vi "Update Data Plot.vi"(6 "Sample Rate (sec/sample)":dbl, 8 "Time interval (s)":i32, 9 "Pump Controller State":T2, 10 "History length (-1; unlimited)":i32=-1, 11 "Graph History Arrays in":T1) -> (0 "Updated Plot History":cluster{timestamp[], dbl[]}[](array[cluster]), 3 "Graph History Arrays out":T1)   [LabVIEW 2020, in "RxnRover.lvlib" / "Pump Controller.lvclass"]
uses:
  Pump Controller.lvclass
  Pump Controller State.ctl
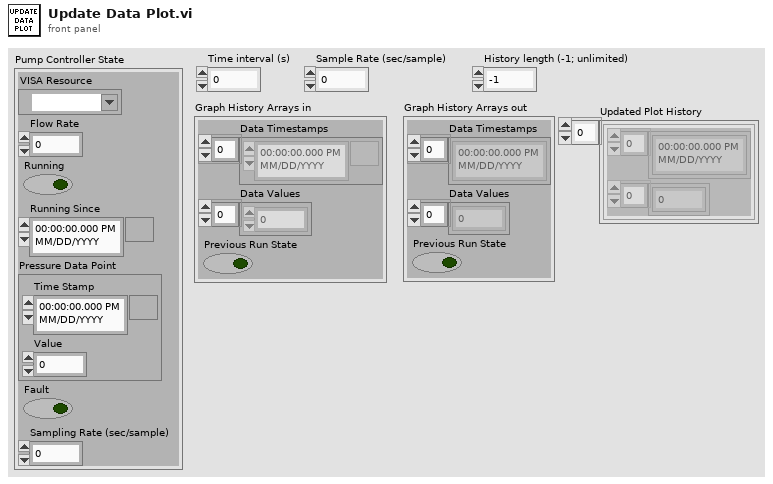
[diagram p1: front panel]
types:
  T1 = cluster{"Data Timestamps":timestamp[], "Data Values":dbl[], "Previous Run State":bool}
  T2 = typedef "RxnRover.lvlib/Pump Controller.lvclass/Pump Controller State.ctl" = cluster{"VISA Resource":refnum<visa-resource-name>, "Flow Rate":dbl, "Running":bool, "Running Since":timestamp, "Pressure Data Point":cluster{"Time Stamp":timestamp, "Value":dbl}, "Fault":bool, "Sampling Rate (sec/sample)":dbl}
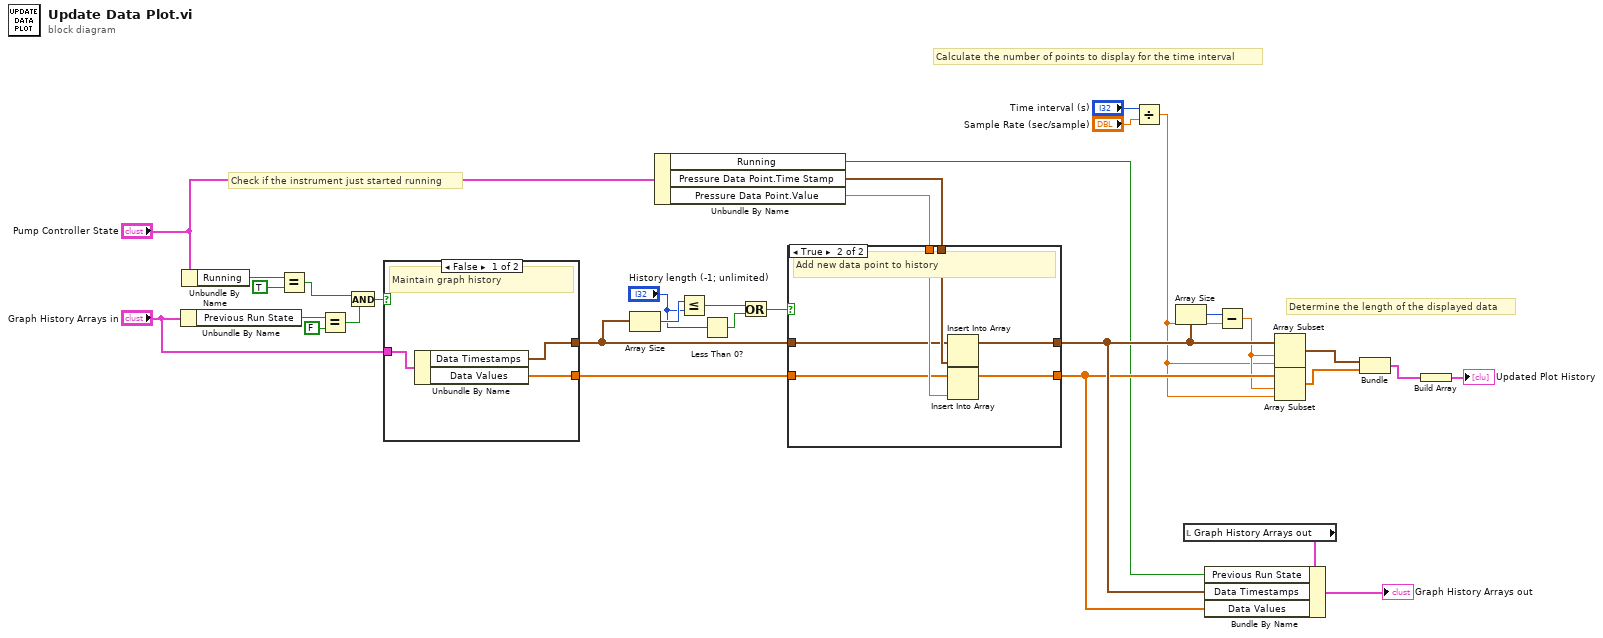
[diagram p0: block diagram]
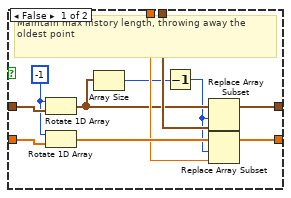
[diagram p2: hidden frame]
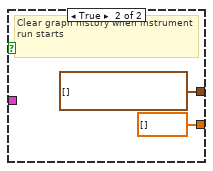
[diagram p3: hidden frame]
diagram:
  # "Check if the instrument just started running"
  # "Calculate the number of points to display for the time interval"
  # "Determine the length of the displayed data"
  n1 = Unbundle By Name("Graph History Arrays in") -> ("Previous Run State"=w19:bool)
  n2 = Unbundle By Name("Pump Controller State") -> ("Running"=w27:bool)
  n3 = Equal?(x=w27, y=TRUE) -> (x = y?=w15:bool)
  n4 = Equal?(x=w19, y=FALSE) -> (x = y?=w16:bool)
  n5 = And(x=w15, y=w16) -> (x .and. y?=w17:bool)
  n6 = case shown="False" w17 {
    tunnel: "Graph History Arrays in" -> [w35 _]
    tunnel: [w34 dbl[] [] ("Data Values")] -> w21
    tunnel: [w33 timestamp[] [] ("Data Timestamps")] -> w8
    frame False {
      # "Maintain graph history"
      n7 = Unbundle By Name(w35) -> ("Data Timestamps"=w33:timestamp[], "Data Values"=w34:dbl[])
    }
    frame True {
      # "Clear graph history when instrument run starts"
    }
  }
  n8 = Array Size(array=w8) -> (size(s)=w7:i32)
  n9 = Unbundle By Name("Pump Controller State") -> ("Running"=w9:bool, "Pressure Data Point.Time Stamp"=w23:timestamp, "Pressure Data Point.Value"=w22:dbl)
  n10 = Less Or Equal?(x=w7, y="History length (-1; unlimited)") -> (x <= y?=w2:bool)
  n11 = Less Than 0?(x="History length (-1; unlimited)") -> (x < 0?=w3:bool)
  n12 = Or(x=w2, y=w3) -> (x .or. y?=w1:bool)
  n13 = case shown="True" w1 {
    tunnel: [w39 w54] -> w26
    tunnel: [w38 w53] -> w25
    tunnel: w23 -> [w43 w52]
    tunnel: w22 -> [w44 w51]
    tunnel: w21 -> [w47 w50]
    tunnel: w8 -> [w48 w49]
    frame False {
      w46 = -1
      # "Maintain max history length, throwing away the oldest point"
      n14 = Rotate 1D Array(1:w48, 2:w46) -> (0:w42:timestamp[])
      n15 = Rotate 1D Array(1:w47, 2:w46) -> (0:w45:dbl[])
      n16 = Array Size(array=w42) -> (size(s)=w41:i32)
      n17 = Decrement(x=w41) -> (x-1=w40:i32)
      n18 = Replace Array Subset(array=w42, new element=w43, index=w40) -> (w39:timestamp[])
      n19 = Replace Array Subset(array=w45, new element=w44, index=w40) -> (w38:dbl[])
    }
    frame True {
      # "Add new data point to history"
      n20 = Insert Into Array(array=w49, new element=w52) -> (w54:timestamp[])  [unwired: 1 in]
      n21 = Insert Into Array(array=w50, new element=w51) -> (w53:dbl[])  [unwired: 1 in]
    }
  }
  n22 = Divide(x="Time interval (s)", y="Sample Rate (sec/sample)") -> (x/y=w13:dbl)
  n23 = Array Size(array=w26) -> (size(s)=w31:i32)
  n24 = local read "Graph History Arrays out"() -> (w24:T1)
  n25 = Bundle By Name(cluster=w24, "Previous Run State"=w9, "Data Timestamps"=w26, "Data Values"=w25) -> (→"Graph History Arrays out":T1)
  n26 = Subtract(x=w31, y=w13) -> (x-y=w14:dbl)
  n27 = Array Subset(array=w26, index=w14, length=w13) -> (w12:timestamp[])
  n28 = Array Subset(array=w25, index=w14, length=w13) -> (w30:dbl[])
  n29 = Bundle(w12, w30) -> (w11:cluster{timestamp[], dbl[]})  [unwired: 1 in]
  n30 = Build Array(w11) -> (→"Updated Plot History":cluster{timestamp[], dbl[]}[])
